vi "SOUR_POW_CORR_COLL_TABL_DATA_A.vi"(0 "VISA IN":refnum<visa-resource-name>, 1 "Cmd 1":i32, 5 "error in":errorcluster, 7 "Channel":i32) -> (14 "VISA Out":refnum<visa-resource-name>, 19 "error out":errorcluster)   [LabVIEW 2018, in "PNA-X.lvlib"]
doc: "SOURce:POWer:CORRection:COLLect:TABLe:DATA \nParameters \n<cnum> Any existing channel number. If unspecified, value is set to 1 \n<char> Choose from: \nNONE - No table selected \nASENsor - Cal Factor table for Power Sensor A \nBSENsor - Cal Factor table for Power Sensor B \nLOSS - Loss compensation table \nExamples SOUR:POW:CORR:COLL:TABL ASEN \nsource1:power2:correction:collect:table:select bsensor \nQuery Syntax SOURce:POWer:CORRection:COLLect:TABLe[:SELect]? \nReturn Type Character \nDefault NONE \nSOURce<cnum>:POWer<port>:CORRection:DATA <data>[,src] \n(Read-Write) Writes and reads source power calibration data. \nWhen querying source power calibration data, if no source power cal data exists for the specified \nchannel and source port, then no data is returned. \nIf a change in the instrument state causes interpolation and/or extrapolation of the source power cal, \nthe correction data associated with this command correspond to the new instrument state (interpolated \nand/or extrapolated data). \nIf the channel is sweeping the source backwards, then the first data point is the highest frequency \nvalue; the last data point is the lowest. Use the SENS:X:VALues? command to return the X-axis \nvalues in the displayed order. \nParameters \n<cnum> Any existing channel number. If unspecified, value is set to 1 \n<port> Port number to correct for source power. If unspecified, value is set to 1. \n<data> Correction Data \n1846\n\n[src] String. (NOT case sensitive). Source port. Optional. Use SOUR:CAT? to \nreturn a list of valid port names. \nWhile this argument can be used to make settings for ALL ports, it is designed \nto access ports that are not simple numbers, such as \"Port 1 Src2\". Otherwise, \nthe <port> argument performs the same function. If both arguments are \nspecified, [src] takes priority. \nExamples SOURce1:POWer2:CORRection:DATA 0.12, -0.34, 0.56 \nQuery Syntax SOURce<cnum>:POWer<port>:CORRection:DATA? [src] \nReturn Type Depends on FORMat:DATA command \nDefault Not Applicable \nSOURce<cnum>:POWer<port>:CORRection:LEVel <num>[,src] \n(Read-Write) Specifies the power level that is expected at the desired reference plane (DUT input or \noutput). This is not used for segment sweep with independent power levels or power sweeps. \nNote: Although this command still works, it is recommended that you specify cal power by setting the \ntest port power and offset value. \nParameters \n<cnum> Any existing channel number. If unspecified, value is set to 1 \n<port> Port number to correct for source power. If unspecified, value is set to 1. \n<num> Cal power level in dBm. Because this could potentially be at the output of a \ndevice-under-test, no limits are placed on this value here. It is realistically \nlimited by the specifications of the device (power sensor) that will be used for \nmeasuring the power. The power delivered to the PNA receiver must never \nexceed PNA specifications for the receiver! \n[src] String. (NOT case sensitive). Source port. Optional. Use SOUR:CAT? to \nreturn a list of valid port names. \nWhile this argument can be used to make settings for ALL ports, it is designed \nto access ports that are not simple numbers, such as \"Port 1 Src2\". Otherwise, \nthe <port> argument performs the same function. If both arguments are \nspecified, [src] takes priority. \nExamples SOUR:POW:CORR:LEV 10 \nsource1:power2:correction:level 0 dbm \nQuery Syntax SOURce:POWer:CORRection:LEVel? [src] \n1847\n\nReturn Type Numeric \nDefault 0 dBm \nSOURce<cnum>:POWer<port>:CORRection:OFFSet[:MAGNitude] <num>[,src] \n(Read-Write) Sets or returns a power level offset from the PNA test port power. This can be a gain or \nloss value (in dB) to account for components you connect between the source and the reference plane \nof your measurement. For example, specify 10 dB to account for a 10 dB amplifier at the input of your \nDUT. \nCal power is the sum of the test port power setting and this offset value. Following the calibration, the \nPNA power readouts are adjusted to the cal power. \nParameters \n<cnum> Any existing channel number. If unspecified, value is set to 1 \n<port> Port number to correct for source power. If unspecified, value is set to 1. \n<num> Gain or loss value in dB. Choose a value between -200 and 200 \n[src] String. (NOT case sensitive). Source port. Optional. Use SOUR:CAT? to \nreturn a list of valid port names. \nWhile this argument can be used to make settings for ALL ports, it is designed \nto access ports that are not simple numbers, such as \"Port 1 Src2\". Otherwise, \nthe <port> argument performs the same function. If both arguments are \nspecified, [src] takes priority. \nExamples SOUR:POW:CORR:OFFS 10 \nsource1:power2:correction:offset:magnitude -3 \nQuery Syntax SOURce:POWer:CORRection:OFFSet[:MAGNitude]? [src] \nReturn Type Numeric \nDefault 0 dB \nSOURce<cnum>:POWer<port>:CORRection[:STATe] <bool>[,src] \n1848\n\n(Read-Write) Enables and disables source power correction for the specified port on the specified \nchannel. \nParameters \n<cnum> Any existing channel number. If unspecified, value is set to 1 \n<port> Port number to correct for source power. If unspecified, value is set to 1. \n<bool> ON (or 1) turns source power correction ON. \nOFF (or 0) - turns source power correction OFF. \n[src] String. (NOT case sensitive). Source port. Optional. Use SOUR:CAT? to return a list \nof valid port names. \nWhile this argument can be used to make settings for ALL ports, it is designed to \naccess ports that are not simple numbers, such as \"Port 1 Src2\". Otherwise, the <port> \nargument performs the same function. If both arguments are specified, [src] takes \npriority. \nExamples SOUR:POW:CORR ON \nsource1:power2:correction:state off \nQuery \nSyntax"
uses:
  PNA-X.lvlib
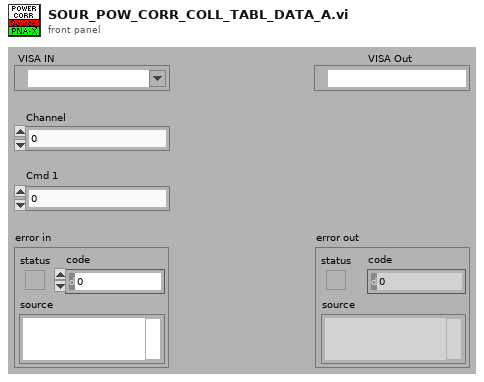
[diagram p1: front panel]
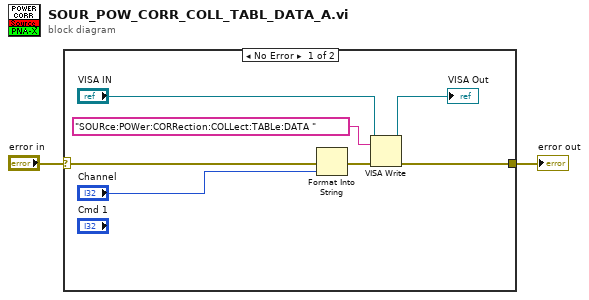
[diagram p0: block diagram]
diagram:
  n1 = case shown="No Error" "error in" {
    selector: "error in" -> [w9 w10]
    tunnel: [w6 w10] -> w1
    frame No Error {
      n2 = Format Into String(error in=w9, "Channel") -> (error out=w8:errorcluster)  [unwired: 2 in, 1 out]
      n3 = VISA Write(VISA resource name="VISA IN", write buffer="SOURce:POWer:CORRection:COLLect:TABLe:DATA " ("Cmdline"), error in (no error)=w8) -> (VISA resource name out=→"VISA Out":refnum<visa-resource-name>, error out=w6:errorcluster)  [unwired: 1 out]
    }
    frame Error {
    }
  }
  "error out" <- w1
